vi "Button Test.vi"(0 "GEA2 Reference In":refnum<k24>, 5 "Test Results In":T1, 11 "Error In":errorcluster) -> (4 "GEA2 Reference Out":refnum<k24>, 6 "Report Text":string, 8 "Pass/Fail?":bool, 15 "Error Out":errorcluster)   [LabVIEW 2016]
doc: "This VI performs the button test. It clears the button press and button history ERDs. Then prompts the user to press all buttons. Then compares the button history value from the ERD to expected response based on hardware type from the config file."
uses:
  C:/Automation/DLLs/PC Dot Net/GeaCommunication.dll
  controls/Test Results.ctl
  Common/LabVIEW GEA2 Toolkit/LabVIEW_GEA2_Toolkit.lvlibp/type defs/Source_Destination.ctl
  Common/LabVIEW GEA2 Toolkit/LabVIEW_GEA2_Toolkit.lvlibp/type defs/ERD Write Data In.ctl
  Common/LabVIEW GEA2 Toolkit/LabVIEW_GEA2_Toolkit.lvlibp/type defs/Data Type.ctl
  Common/LabVIEW GEA2 Toolkit/LabVIEW_GEA2_Toolkit.lvlibp/type defs/ERD Read Data In.ctl
  Common/LabVIEW GEA2 Toolkit/LabVIEW_GEA2_Toolkit.lvlibp
panel:
  out "Test Results Out":T1
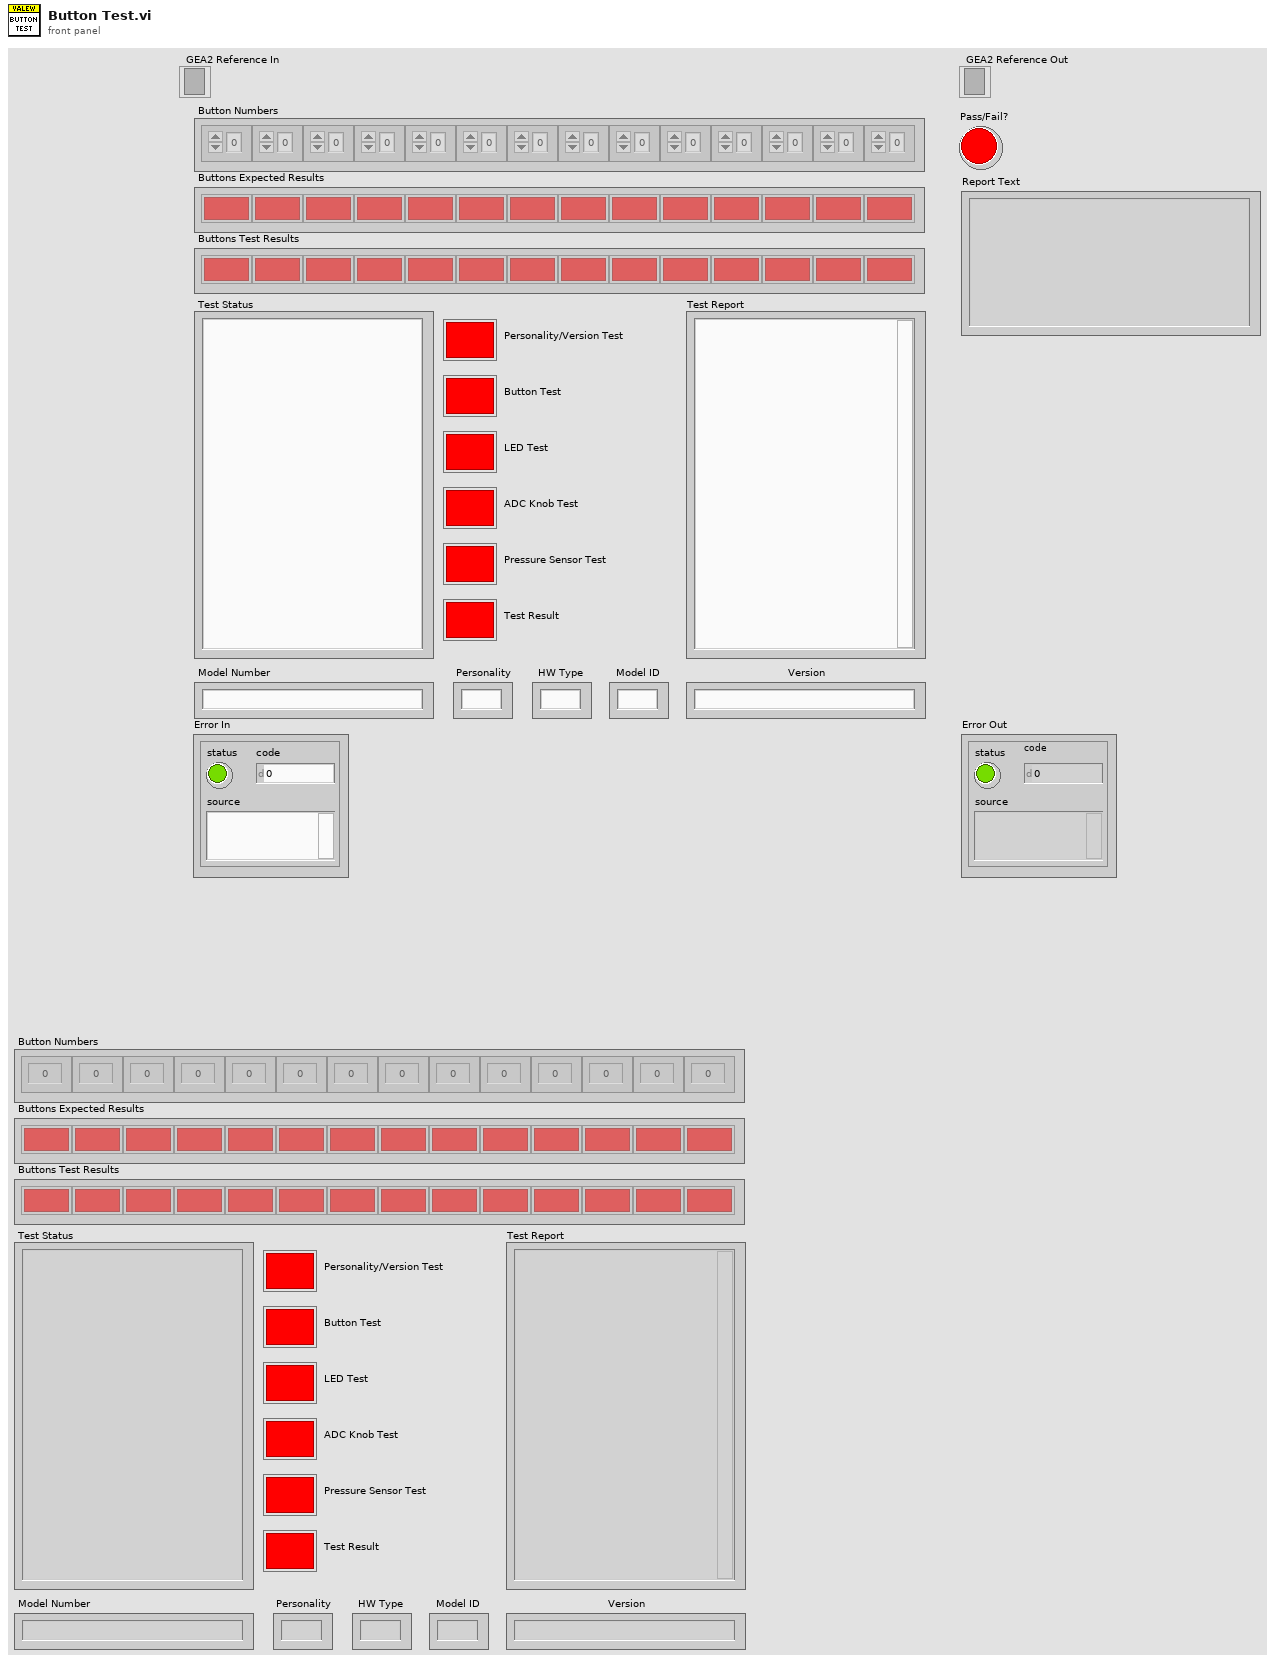
[diagram p1: front panel]
types:
  T1 = typedef "Test Results.ctl" = cluster{"Test Status":string, "Personality/Version Test ":bool, "Test Report":string, "Model Number":string, "Button Numbers":i32[], "Buttons Test Results":bool[], "Buttons Expected Results":bool[], "Model ID":string, "Personality":string, "HW Type":string, "Version":string, "Button Test":bool, "LED Test":bool, "ADC Knob Test":bool, "Pressure Sensor Test":bool, "Test Result":bool}
  T2 = typedef "LabVIEW_GEA2_Toolkit.lvlibp/Source_Destination.ctl" = cluster{"Source":u8, "Destination":u8}
  T3 = typedef "LabVIEW_GEA2_Toolkit.lvlibp/ERD Read Data In.ctl" = cluster{"ERD Number":u16, "Data Type":T4}
  T4 = typedef "LabVIEW_GEA2_Toolkit.lvlibp/Data Type.ctl" = enum16{"string", "boolean", "uint8_t", "uint16_t", "uint32_t", "uint64_t", "int8_t", "int16_t", "int32_t", "int64_t"}
  T5 = typedef "LabVIEW_GEA2_Toolkit.lvlibp/ERD Write Data In.ctl" = cluster{"ERD Number":u16, "Data Type":T4, "Data":string}
  T6 = typedef "LabVIEW_GEA2_Toolkit.lvlibp/ERD Read Data Out.ctl" = cluster{"ERD Number":u16, "Data":string}
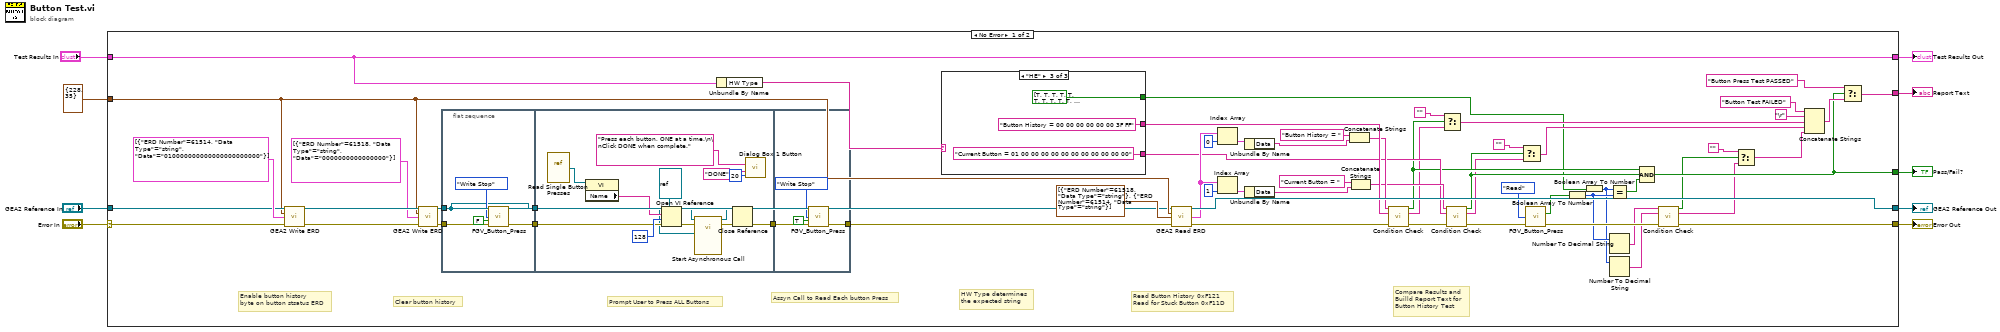
[diagram p0: block diagram]
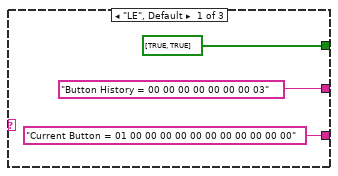
[diagram p2: hidden frame]
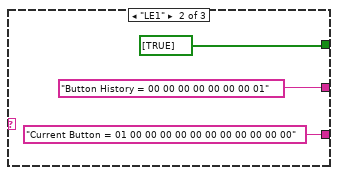
[diagram p3: hidden frame]
diagram:
  n1 = case shown="No Error" "Error In" {
    selector: "Error In" -> [w56 w103]
    tunnel: "GEA2 Reference In" -> [w66 w104]
    tunnel: [w62 w104] -> w8
    tunnel: T2 {"Source"=228, "Destination"=35} ("GEA Inputs") -> [w61 _]
    tunnel: [w59 _] -> w6
    tunnel: [w20 w103] -> w5
    tunnel: [w51 _] -> w4
    tunnel: "Test Results In" -> [w53 _]
    tunnel: [w53 _] -> w1
    frame No Error {
      # "Assyn Call to Read Each button Press"
      # "Compare Results and \nBuilld Report Text for \nButton History Test"
      # "HW Type determines\nthe expected string"
      # "Prompt User to Press ALL Buttons"
      # "Read Button History 0xF121\nRead for Stuck Button 0xF11D"
      # "Clear button history"
      # "Enable button history\nbyte on button stsatus ERD"
      n2 = call "GEA2 Write ERD.vi"("GEA2 Reference In"=w66, "GEA Inputs"=w61, "Write ERD List"=T5[] [{"ERD Number"=61514, "Data Type"=enum."string", "Data"="010000000000000000000000"}], "Error In"=w56) -> ("GEA2 Reference Out"=w68:refnum<k24>, "Error Out"=w69:errorcluster)  [unwired: 9 in, 1 out]
      n3 = call "GEA2 Write ERD.vi"("GEA2 Reference In"=w68, "GEA Inputs"=w61, "Write ERD List"=T5[] [{"ERD Number"=61518, "Data Type"=enum."string", "Data"="0000000000000000"}], "Error In"=w69) -> ("GEA2 Reference Out"=w28:refnum<k24>, "Error Out"=w65:errorcluster)  [unwired: 9 in, 1 out]
      n4 = flat-sequence {
        tunnel: w28 -> [w81]
        tunnel: w65 -> [w83]
        tunnel: [w82] -> w11
        tunnel: [w81] -> w10
        tunnel: [w93] -> w29
        tunnel: w11 -> [w94]
        tunnel: w10 -> [w86]
        tunnel: [w101] -> w27
        tunnel: w29 -> [w102]
        frame #0 {
          n5 = call "FGV_Button_Press.vi"("Action"=enum16{"Read", "Write Stop", "Write Result"}."Write Stop", "Boolean In"=FALSE ("Boolean 2"), "Error In"=w83) -> ("Error Out"=w82:errorcluster)  [unwired: 10 in, 2 out]
        }
        frame #1 {
          n6 = vi-ref "Read Single Button Presses.vi"() -> (w91:refnum<vi>)
          n7 = property class="VI"(reference=w91) -> ("Name"=w92:string)  [unwired: 1 in, 2 out]
          n8 = Open VI Reference(type specifier VI Refnum (for type only)=refnum<vi> refnum, vi path=w92, options=128, error in (no error)=w94) -> (vi reference=w87:refnum<vi>, error out=w90:errorcluster)  [unwired: 2 in]
          n9 = call-by-ref "Start Asynchronous Call"(reference=w87, error in=w90, "GEA2 Reference In"=w86) -> (reference out=w85:refnum<vi>, error out=w89:errorcluster)  [unwired: 12 in, 3 out]
          n10 = Close Reference(reference=w85, error in (no error)=w89) -> (error out=w93:errorcluster)
          n11 = call "Dialog Box 1 Button.vi"("Input"="Press each button, ONE at a time.\n\nClick DONE when complete.", "Button Name (\"OK\")"="DONE" ("Button Name (\"OK\")"), "Font Size"=u32 20) -> ()  [unwired: 13 in]
        }
        frame #2 {
          n12 = call "FGV_Button_Press.vi"("Action"=enum16{"Read", "Write Stop", "Write Result"}."Write Stop", "Boolean In"=TRUE ("Boolean 2"), "Error In"=w102) -> ("Error Out"=w101:errorcluster)  [unwired: 10 in, 2 out]
        }
      }
      n13 = Unbundle By Name(w53) -> ("HW Type"=w52:string)
      n14 = case shown="\"HE\"" w52 {
        tunnel: ["Button History = 00 00 00 00 00 00 00 03" "Button History = 00 00 00 00 00 00 00 01" "Button History = 00 00 00 00 00 00 3F FF"] -> w45
        tunnel: ["Current Button = 01 00 00 00 00 00 00 00 00 00 00 00" "Current Button = 01 00 00 00 00 00 00 00 00 00 00 00" "Current Button = 01 00 00 00 00 00 00 00 00 00 00 00"] -> w38
        tunnel: [bool[] [TRUE, TRUE] ("Boolean Array Out") bool[] [TRUE] ("Boolean Array Out") bool[] [TRUE, TRUE, TRUE, TRUE, TRUE, TRUE, TRUE, TRUE, TRUE, TRUE, TRUE, TRUE, TRUE, TRUE] ("Boolean Array Out")] -> w24
        frame "LE", Default {
        }
        frame "LE1" {
        }
        frame "HE" {
        }
      }
      n15 = call "GEA2 Read ERD.vi"("GEA2 Reference In"=w28, "GEA Inputs"=w61, "Read ERD List"=T3[] [{"ERD Number"=61518, "Data Type"=enum."string"}, {"ERD Number"=61514, "Data Type"=enum."string"}], "Error In"=w27) -> ("GEA2 Reference Out"=w62:refnum<k24>, "ERD Data Out"=w49:T6[], "Error Out"=w58:errorcluster)  [unwired: 8 in, 1 out]
      n16 = Index Array(array=w49, index=0) -> (element=w63:T6)
      n17 = Index Array(array=w49, index=1) -> (element=w46:T6)
      n18 = Unbundle By Name(w63) -> ("Data"=w43:string)
      n19 = Unbundle By Name(w46) -> ("Data"=w40:string)
      n20 = Concatenate Strings("Button History = ", w43) -> (w42:string)
      n21 = Concatenate Strings("Current Button = ", w40) -> (w39:string)
      n22 = call "Condition Check.vi"("Actual"=w42, "Low"=w45, "Error In"=w58) -> ("Pass/Fail"=w36:bool, "Report Text"=w35:string, "Error Out"=w50:errorcluster)  [unwired: 10 in]
      n23 = Select(t="", s=w36, f=w35) -> (s? t:f=w34:string)
      n24 = call "Condition Check.vi"("Actual"=w39, "Low"=w38, "Error In"=w50) -> ("Pass/Fail"=w32:bool, "Report Text"=w31:string, "Error Out"=w26:errorcluster)  [unwired: 10 in]
      n25 = Select(t="", s=w32, f=w31) -> (s? t:f=w30:string)
      n26 = call "FGV_Button_Press.vi"("Action"=enum16{"Read", "Write Stop", "Write Result"}."Read", "Error In"=w26) -> ("Boolean Array Out"=w25:bool[], "Error Out"=w21:errorcluster)  [unwired: 11 in, 1 out]
      n27 = Boolean Array To Number(Boolean array=w25) -> (number=w18:u32)
      n28 = Boolean Array To Number(Boolean array=w24) -> (number=w16:u32)
      n29 = Number To Decimal String(number=w18) -> (decimal integer string=w17:string)  [unwired: 1 in]
      n30 = Equal?(x=w16, y=w18) -> (x = y?=w23:bool)
      n31 = Number To Decimal String(number=w16) -> (decimal integer string=w15:string)  [unwired: 1 in]
      n32 = Compound Arithmetic op=AND(w36, w32, w23) -> (w51:bool)
      n33 = call "Condition Check.vi"("Actual"=w17, "Low"=w15, "Error In"=w21) -> ("Pass/Fail"=w14:bool, "Report Text"=w13:string, "Error Out"=w20:errorcluster)  [unwired: 10 in]
      n34 = Select(t="", s=w14, f=w13) -> (s? t:f=w12:string)
      n35 = Concatenate Strings("Button Test FAILED" ("string"), "\r", w34, w30, w12) -> (w57:string)
      n36 = Select(t="Button Press Test PASSED", s=w51, f=w57) -> (s? t:f=w59:string)
    }
    frame Error {
    }
  }
  "Error Out" <- w5
  "GEA2 Reference Out" <- w8
  "Pass/Fail?" <- w4
  "Report Text" <- w6
  "Test Results Out" <- w1
